vi "Orca Flash Capture Set Auto Waveform.vi"(0 "Interline Interval":dbl, 2 "Filter Index":i32, 7 "Waveform Parameters":dbl[](array[numeric]), 11 "Filter Offsets":dbl[](array[numeric])) -> (4 "Offset (V)":dbl, 6 "Amplitude (V)":dbl, 8 "Samples per Channel":i32, 10 "Delay (ms)":dbl, 13 "Line Scan Settings":T1)   [LabVIEW 2016]
uses:
  Orca Flash Capture Manager Controls/Orca Flash Capture Line Scan Settings.ctl
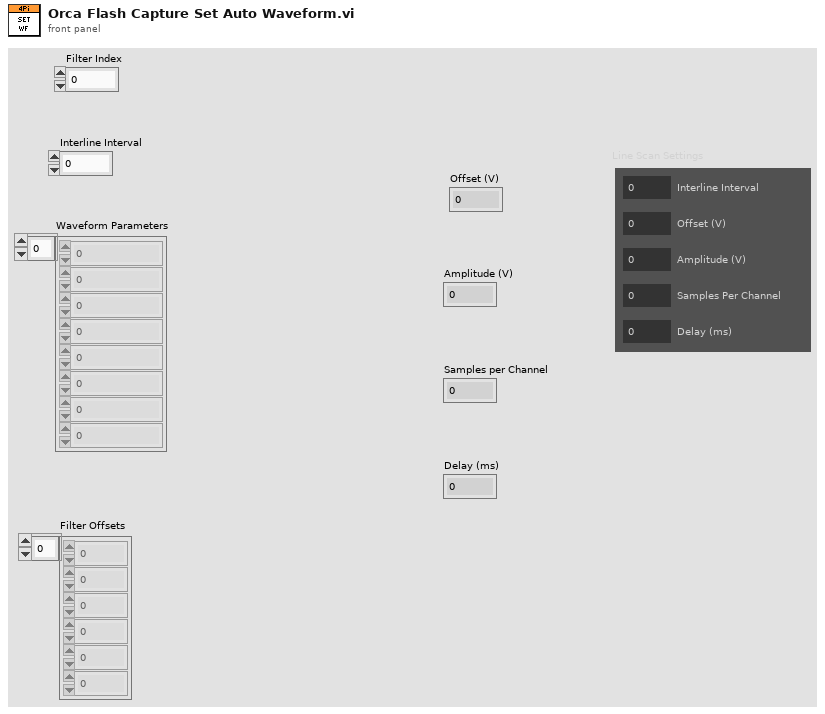
[diagram p1: front panel]
types:
  T1 = typedef "Orca Flash Capture Line Scan Settings.ctl" = cluster{"Interline Interval":dbl, "Offset (V)":dbl, "Amplitude (V)":dbl, "Samples Per Channel":dbl, "Delay (ms)":dbl}
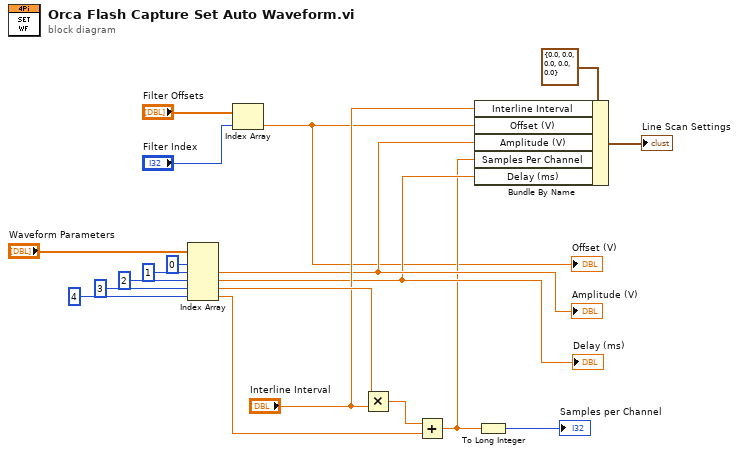
[diagram p0: block diagram]
diagram:
  n1 = Index Array(array="Waveform Parameters", index #1=0 ("index"), index #2=1 ("index"), index #3=2 ("index"), index #4=3 ("index"), index #5=4 ("index")) -> (element #2=w7:dbl, element #3=w6:dbl, element #4=w13:dbl, element #5=w11:dbl)  [unwired: 1 out]
  "Amplitude (V)" <- w7
  "Delay (ms)" <- w6
  n2 = Index Array(array="Filter Offsets", index="Filter Index") -> (element=w1:dbl)
  "Offset (V)" <- w1
  n3 = Multiply(x=w13, y="Interline Interval") -> (x*y=w12:dbl)
  n4 = Add(x=w12, y=w11) -> (x+y=w5:dbl)
  n5 = Bundle By Name(cluster=T1 {"Interline Interval"=0.0, "Offset (V)"=0.0, "Amplitude (V)"=0.0, "Samples Per Channel"=0.0, "Delay (ms)"=0.0} ("Line Scan Settings"), "Interline Interval"="Interline Interval", "Offset (V)"=w1, "Amplitude (V)"=w7, "Samples Per Channel"=w5, "Delay (ms)"=w6) -> (→"Line Scan Settings":T1)
  n6 = To Long Integer(number=w5) -> (32bit integer=→"Samples per Channel":i32)
